vi "HFRR ADV v05.vi"() -> ()   [LabVIEW 2025] (continued)
      tunnel: w686 -> [w706 w859]
      tunnel: [w705 _] -> _
      frame No Error {
        n460 = stacked-sequence {
          tunnel: w706 -> [w730 _]
          tunnel: w702 -> [w729 _]
          tunnel: [w716 _] -> w705
          tunnel: [w715 _] -> w704
          tunnel: [w714 _] -> w703
          frame #0 {
            n461 = property class="Instr"(reference=w730, error in=w729) -> (reference out=w713:refnum<visa-resource-name>, error out=w728:errorcluster, "Serial Settings:Number of Bytes at Serial Port"=w709:u32)
            "Port 2" <- w709
            n462 = Greater?(x=w709, y=u32 23) -> (0:w711:bool)
            n463 = Not(x=w711) -> ()  [unwired: 1 out]
            n464 = case shown="True" w711 {
              tunnel: w713 -> [w745 w770]
              tunnel: w728 -> [w744 w771]
              tunnel: [w744 w773] -> w724
              tunnel: [w745 w772] -> w725
              frame False {
              }
              frame True {
                # "Out as Volts"
                n465 = local read "Residual Due"() -> (w769:string)
                n466 = while {
                  tunnel: [w813] -> w773
                  tunnel: [w812] -> w772
                  tunnel: w771 -> [w811]
                  tunnel: w770 -> [w810]
                  tunnel: [w807] -> _
                  shift-right: [w805] -> w768
                  shift-left: w769 -> [w804]
                  i -> [w807]
                  stop <- w808 stop-if-true
                  n467 = property class="Instr"(reference=w810, error in=w811) -> (reference out=w815:refnum<visa-resource-name>, error out=w814:errorcluster, "Serial Settings:Number of Bytes at Serial Port"=w806:u32)
                  n468 = VISA Read(VISA resource name=w815, byte count=w806, error in (no error)=w814) -> (VISA resource name out=w812:refnum<visa-resource-name>, read buffer=w803:string, error out=w813:errorcluster)  [unwired: 1 out]
                  n469 = Greater?(x=w806, y=u32 8) -> (0:w808:bool)
                  n470 = Concatenate Strings(w804, w803) -> (w805:string)
                }
                n471 = while {
                  shift-right: [w796] -> w752
                  shift-left: w768 -> [w801]
                  tunnel: [w795] -> w764 mode=indexing
                  tunnel: [w794] -> _
                  i -> [w794]
                  stop <- w798 stop-if-true
                  n472 = Match Pattern(string=w801, regular expression="*") -> (after substring=w799:string)  [unwired: 1 in, 3 out]
                  n473 = Match Pattern(string=w799, regular expression="&") -> (before substring=w795:string, after substring=w796:string, offset past match=w797:i32)  [unwired: 1 in, 1 out]
                  n474 = Less Than 0?(x=w797) -> (x < 0?=w798:bool)
                }
                n475 = Array Size(array=w764) -> (size(s)=w767:i32)
                n476 = local write "Residual Due"(w752) -> ()
                n477 = Decrement(x=w767) -> (x-1=w765:i32)
                n478 = Delete From Array(array=w764, length=1, index=w765) -> (array with subset deleted=w763:string[])  [unwired: 1 out]
                n479 = Array Size(array=w763) -> (size(s)=w751:i32)
                n480 = Decrement(x=w751) -> (x-1=w750:i32)
                n481 = while {
                  tunnel: w763 -> [w782] mode=indexing
                  tunnel: w750 -> [w781]
                  tunnel: [w779] -> w758 mode=indexing
                  tunnel: [w778] -> w757 mode=indexing
                  tunnel: [w777] -> w756 mode=indexing
                  tunnel: [w776] -> w755 mode=indexing
                  tunnel: [w775] -> w753 mode=indexing
                  tunnel: [w774] -> _
                  i -> [w774]
                  stop <- w780 stop-if-true
                  w791 = u32 0 ("length (rest)")
                  w790 = ";" ("regular expression")
                  n482 = Less Or Equal?(x=w781, y=w774) -> (x <= y?=w780:bool)
                  n483 = Match Pattern(string=w782, regular expression=w790) -> (before substring=w783:string, after substring=w784:string)  [unwired: 1 in, 2 out]
                  n484 = Match Pattern(string=w784, regular expression=w790) -> (before substring=w787:string, after substring=w785:string)  [unwired: 1 in, 2 out]
                  n485 = Decimal String To Number(string=w783, default (0L)=w791) -> (number=w779:u32)  [unwired: 1 in, 1 out]
                  n486 = Decimal String To Number(string=w787, default (0L)=w791) -> (number=w778:u32)  [unwired: 1 in, 1 out]
                  n487 = Match Pattern(string=w785, regular expression=w790) -> (before substring=w788:string, after substring=w786:string)  [unwired: 1 in, 2 out]
                  n488 = Decimal String To Number(string=w788, default (0L)=w791) -> (number=w777:u32)  [unwired: 1 in, 1 out]
                  n489 = Match Pattern(string=w786, regular expression=w790) -> (before substring=w789:string, after substring=w793:string)  [unwired: 1 in, 2 out]
                  n490 = Decimal String To Number(string=w789, default (0L)=w791) -> (number=w776:u32)  [unwired: 1 in, 1 out]
                  n491 = Decimal String To Number(string=w793, default (0L)=u8 0 ("length (rest)")) -> (number=w775:u8)  [unwired: 1 in, 1 out]
                }
                "Din" <- w753
                n492 = Bundle(w758, w757, w756, w755) -> (w760:cluster{u32[], u32[], u32[], u32[]})  [unwired: 1 in]
                n493 = Divide(x=w760, y=4095 ("length (rest)")) -> (x/y=w762:cluster{dbl[], dbl[], dbl[], dbl[]})
                n494 = Multiply(x=w762, y=sgl 3.32 ("Numeric")) -> (x*y=w754:cluster{dbl[], dbl[], dbl[], dbl[]})
                n495 = Unbundle(w754) -> (→"ECR":dbl[], →"Rtemp":dbl[], →"Air temp":dbl[], →"Ch3 2":dbl[])
              }
            }
            n496 = call "Elapsed Time10"("Time Target (s)"=2.0, "Reset"=w711, "Auto Reset"=FALSE) -> ("Time has Elapsed"=→"Port 2a":bool)  [unwired: 9 in, 7 out]
            n497 = local read "Due Com"() -> (w717:string[])
            n498 = Array Size(array=w717) -> (size(s)=w716:i32)
            n499 = Delete From Array(array=w717, length=1, index=0) -> (deleted portion=w720:string[], array with subset deleted=w721:string[])
            n500 = local write "Due Com"(w721) -> ()
            n501 = Index Array(array=w720, index=0) -> (element=w718:string)
            n502 = Not Equal?(x=w718, y="") -> (x != y?=w726:bool)
            n503 = case shown="True" w726 {
              tunnel: w725 -> [w732 w737]
              tunnel: [w732 w741] -> w715
              tunnel: w724 -> [w731 w736]
              tunnel: [w731 w739] -> w714
              tunnel: w718 -> [_ w735]
              tunnel: [_ w738] -> _
              frame False {
                # "DATA  WRITE LOOP"
              }
              frame True {
                n504 = Concatenate Strings(w735, "\r\n") -> (w734:string)
                n505 = VISA Write(VISA resource name=w737, write buffer=w734, error in (no error)=w736) -> (VISA resource name out=w741:refnum<visa-resource-name>, return count=w738:u32, error out=w740:errorcluster)
                n506 = flat-sequence {
                  tunnel: w740 -> [w742]
                  tunnel: [w742] -> w739
                  frame #0 {
                    n507 = Wait (ms)(milliseconds to wait=u32 5) -> ()  [unwired: 1 out]
                  }
                }
              }
            }
          }
          frame #1 {
            w824 = 10 ("y")
            w829 = 10 ("y")
            n508 = local read "Rtemp"() -> (w817:dbl[])
            n509 = local read "ecr buf"() -> (w818:dbl[])
            n510 = for {
              tunnel: w817 -> [w841] mode=indexing
              shift-right: [w842] -> w825
              shift-left: dbl[] [] ("temp buf 2") -> [w843]
              n511 = Build Array (concatenate)(w843, w841) -> (w844:dbl[])
              n512 = Equal To 0?(x=w841) -> (x = 0?=w845:bool)
              n513 = Select(t=w843, s=w845, f=w844) -> (s? t:f=w842:dbl[])
            }
            n514 = local read "ECR"() -> (w816:dbl[])
            n515 = Insert Into Array(array=w816, index=0, new element=w818) -> (w822:dbl[])
            n516 = local read "temp buf"() -> (w826:dbl[])
            n517 = Array Size(array=w822) -> (size(s)=w823:i32)
            n518 = Greater?(x=w823, y=w824) -> (0:w821:bool)
            n519 = case shown="True" w821 {
              tunnel: w822 -> [w834 w840]
              tunnel: w823 -> [_ w838]
              tunnel: w824 -> [_ w837]
              tunnel: [w834 w835] -> w819
              frame False {
              }
              frame True {
                n520 = Subtract(x=w838, y=w837) -> (x-y=w836:i32)
                n521 = Delete From Array(array=w840, length=w836, index=0) -> (array with subset deleted=w835:dbl[])  [unwired: 1 out]
              }
            }
            "ecr buf" <- w819
            n522 = Insert Into Array(array=w825, index=0, new element=w826) -> (w831:dbl[])
            n523 = Array Size(array=w831) -> (size(s)=w830:i32)
            n524 = Greater?(x=w830, y=w829) -> (0:w832:bool)
            n525 = case shown="True" w832 {
              tunnel: w831 -> [w846 w852]
              tunnel: w830 -> [_ w850]
              tunnel: w829 -> [_ w849]
              tunnel: [w846 w847] -> w828
              frame False {
              }
              frame True {
                n526 = Subtract(x=w850, y=w849) -> (x-y=w848:i32)
                n527 = Delete From Array(array=w852, length=w848, index=0) -> (array with subset deleted=w847:dbl[])  [unwired: 1 out]
              }
            }
            "temp buf" <- w828
          }
        }
      }
      frame Error {
        w867 = u16 0 items=["None", "XON/XOFF", "RTS/CTS", "XON/XOFF & RTS/CTS", "DTR/DSR", "XON/XOFF & DTR/DSR"] ("flow control (0:none)  2")
        w865 = u16 10 items=["1.0"=10, "1.5"=15, "2.0"=20] ("stop bits 2")
        w863 = u16 0 items=["None", "Odd", "Even", "Mark", "Space"] ("parity 2")
        w864 = u32 10000  # timeout (10sec)
        n528 = VISA Clear(VISA resource name=w859, error in (no error)=w856) -> (VISA resource name out=w858:refnum<visa-resource-name>, error out=w857:errorcluster)
        n529 = VISA Close(VISA resource name=w858, error in (no error)=w857) -> (error out=w860:errorcluster)
        n530 = call <vilib>:"Clear Errors.vi"("error in (no error)"=w860) -> ()  [unwired: 5 in, 2 out]
        n531 = local read "Com Port 2"() -> (w853:refnum<visa-resource-name>)
        "visa due" <- w853
        n532 = call-poly "VISA Configure Serial Port"("VISA resource name"=w853, "timeout (10sec)"=w864, "baud rate (9600)"=u32 250000 ("baud rate  2"), "data bits (8)"=u16 8 ("data bits  2"), "parity (0:none)"=w863, "stop bits (10: 1 bit)"=w865, "flow control (0:none)"=w867) -> ("VISA resource name out"=w868:refnum<visa-resource-name>, "error out"=w869:errorcluster)  [unwired: 7 in]
        n533 = flat-sequence {
          tunnel: w868 -> [w871]
          tunnel: w869 -> [w870]
          tunnel: [w871] -> w861
          tunnel: [w870] -> w854
          frame #0 {
            n534 = Wait (ms)(milliseconds to wait=u32 50) -> ()  [unwired: 1 out]
          }
        }
        "Residual Due" <- ""
        "Port 2 Error" <- w854
      }
    }
    n535 = local read "Quit"() -> (w680:bool)
    "Error Due" <- w688
  }
  n536 = property on="RUN" class="Bool (strict)"("Visible"=TRUE) -> ()  [unwired: 2 in, 2 out]
  n537 = while {
    tunnel: [w889] -> _
    tunnel: [w873] -> w38
    i -> [w889]
    stop <- w873 stop-if-true
    n538 = local read "conststatus"() -> (w877:dbl)
    n539 = local read "Main Tab"() -> (w875:T2)
    n540 = local read "EDIT"() -> (w895:bool)
    n541 = local read "Rate"() -> (w894:dbl)
    n542 = case shown="True" w895 {
      tunnel: [FALSE TRUE] -> w881
      frame False {
      }
      frame True {
      }
    }
    n543 = property on="Time slide" class="Slide (strict)"("Scale.Range:Maximum"=2500.0) -> ()  [unwired: 2 in, 2 out]
    n544 = Equal?(x=w875, y=T15."About" ("Main Tab")) -> (x = y?=w887:bool)
    n545 = Equal?(x=w877, y=0.0) -> (x = y?=w878:bool)
    n546 = Divide(x=1.0, y=w894) -> (x/y=w890:dbl)
    "Time 2" <- w890
    n547 = case shown="True" w878 {
      frame False {
      }
      frame True {
        # "C:\\WinDucom\\calibrate WO 2391.dcf"
        n548 = local write "Lan flag"(22) -> ()
        n549 = local write "conststatus"(10.0 ("rpm value : 2")) -> ()
        n550 = String To Path(string="C:\\LAB-IQ-NXT\\calibrate WO 2464.dcf") -> (path=w901:path)
        n551 = Open/Create/Replace File "Open File"(file path (use dialog)=w901) -> (refnum out=w899:refnum<file>)  [unwired: 5 in, 2 out]
        n552 = for {
          N: 23 -> [_]
          tunnel: w899 -> [w910]
          i -> [w904]
          (unwired) TRUE ("line mode (F)")
          n553 = Read from Text File "Read File"(file (use dialog)=w910) -> (text=w909:string)  [unwired: 3 in, 3 out]
          n554 = Match Pattern(string=w909, regular expression="]") -> (after substring=w907:string)  [unwired: 1 in, 3 out]
          n555 = String Subset(string=w909, offset (0)=5, length (rest)=10 ("length (rest)")) -> (substring=w902:string)
          n556 = Fract/Exp String To Number(string=w902) -> (number=w903:dbl)  [unwired: 3 in, 1 out]
          n557 = Match Pattern(string=w907, regular expression="-") -> (before substring=w905:string)  [unwired: 1 in, 3 out]
          n558 = case shown="18" w904 {
            tunnel: w903 -> [w913 w914 w915 w916 _ _ _ w921 w922 w923 w926 w927 w928 w929 w930 w931 w932 w935 w936 _ _ w939 _ _]
            tunnel: w905 -> [_ _ _ _ w917 w918 w919 _ _ _ _ _ _ _ _ _ _ _ _ w937 w938 _ w940 _]
            frame 0 {
              n559 = local write "FRIC. FORCE :"(w913) -> ()
            }
            frame 1 {
              n560 = local write "TEMPERATURE :"(w914) -> ()
            }
            frame 2 {
              n561 = local write "HUMIDITY:"(w915) -> ()
            }
            frame 3 {
              n562 = local write "AIR TEMPERATURE :"(w916) -> ()
            }
            frame 4 {
              n563 = local write "Com Port 1"(w917) -> ()
            }
            frame 5 {
              n564 = local write "Com Port 2"(w918) -> ()
              n565 = local write "visa due"(w918) -> ()
            }
            frame 6 {
              n566 = String To Path(string=w919) -> (path=w920:path)
              n567 = local write "File Path"(w920) -> ()
              "String" <- w919
            }
            frame 7 {
              n568 = local write "DISPLACEMENT :"(w921) -> ()
            }
            frame 8 {
              n569 = local write "STROKE GAIN :"(w922) -> ()
            }
            frame 9 {
              n570 = local read "Stroke PID Gains"() -> (w925:T8)
              n571 = Bundle By Name(cluster=w925, "Proportional Gain (Kc)"=w923) -> (w924:T8)
              n572 = local write "Stroke PID Gains"(w924) -> ()
            }
            frame 10 {
              n573 = local write "Language Selection"(w926) -> ()
            }
            frame 11 {
              n574 = local write "CH-POWER +"(w927) -> ()
            }
            frame 12 {
              n575 = local write "CH-POWER -"(w928) -> ()
            }
            frame 13 {
              n576 = local write "CH-HEATER"(w929) -> ()
            }
            frame 14 {
              n577 = local write "CH-HUMIDITY WET"(w930) -> ()
            }
            frame 15 {
              n578 = local write "CH-HUMIDITY DRY"(w931) -> ()
            }
            frame 16 {
              n579 = local read "Stroke PID Gains"() -> (w934:T8)
              n580 = Bundle By Name(cluster=w934, "Integral Time (Ti, min)"=w932) -> (w933:T8)
              n581 = local write "Stroke PID Gains"(w933) -> ()
            }
            frame 17 {
              n582 = local write "AIR TEMP INTERCEPT:"(w935) -> ()
            }
            frame 18 {
              n583 = local write "TEMP INTERCEPT:"(w936) -> ()
            }
            frame 19 {
              n584 = local write "S.NO"(w937) -> ()
            }
            frame 20 {
              n585 = local write "Com Port 3"(w938) -> ()
            }
            frame 21 {
              n586 = local write "LvdtOff"(w939) -> ()
            }
            frame 22 {
              n587 = local write "Humidity"(w940) -> ()
            }
            frame 23, Default {
            }
          }
        }
      }
    }
    n588 = Select(t=u32 2500 ("milliseconds to wait"), s=w887, f=u32 500 ("milliseconds to wait")) -> (s? t:f=w885:u32)
    n589 = Multiply(x=w890, y=w885) -> (x*y=w892:dbl)
    n590 = property on="FF Calibration g" class="WFGraph (strict)"("Visible"=w881) -> ()  [unwired: 2 in, 2 out]
    n591 = property on="Lift" class="Bool (strict)"("Visible"=w881) -> ()  [unwired: 2 in, 2 out]
    n592 = property on="Threshold" class="DigNum (strict)"("Visible"=w881) -> ()  [unwired: 2 in, 2 out]
    n593 = property on="Time slide" class="Slide (strict)"("Visible"=w881) -> ()  [unwired: 2 in, 2 out]
    n594 = call "Elapsed Time2"("Time Target (s)"=w892, "Auto Reset"=TRUE) -> ("Time has Elapsed"=w882:bool)  [unwired: 10 in, 7 out]
    n595 = case shown="True" w882 {
      frame False {
        # "79.77669138"
        # "2.3554"
        n596 = local read "FRIC. FORCE :"() -> (w945:dbl)
        n597 = local read "FF cal val"() -> (w942:dbl[])
        n598 = Multiply(x=w945, y=79.77669138) -> (x*y=w944:dbl)
        n599 = Multiply(x=w942, y=w944) -> (x*y=→"FF Calibration g":dbl[])
        "Err Count" <- 0 ("y")
      }
      frame True {
        n600 = stacked-sequence {
          frame #0 {
            n601 = stacked-sequence {
              frame #0 {
                "Lift" <- TRUE ("Lift")
              }
            }
          }
          frame #1 {
            w957 = 2500 ("y")
            n602 = local read "RUN"() -> (w949:bool)
            n603 = local read "FF1"() -> (w952:dbl[])
            n604 = case shown="False" w949 {
              frame False {
                n605 = local write "Frequency"(0.0 ("Frequency")) -> ()
              }
              frame True {
              }
            }
            n606 = Array Size(array=w952) -> (size(s)=w951:i32)
            n607 = local read "Ch1"() -> (w948:dbl[])
            "Waveform Chart 2" <- w948
            n608 = call-poly <vilib>:"Mean.vi"("X"=w948) -> ("mean"=→"Raw Mean":dbl)  [unwired: 1 out]
            n609 = Insert Into Array(array=w952, index=w951, new element=w948) -> (w954:dbl[])
            n610 = Array Size(array=w954) -> (size(s)=w958:i32)
            n611 = Subtract(x=w958, y=w957) -> (x-y=w956:i32)
            n612 = Greater?(x=w958, y=w957) -> (0:w959:bool)
            n613 = case shown="True" w959 {
              tunnel: w956 -> [_ w963]
              tunnel: [w961 w965] -> w950
              tunnel: w954 -> [w961 w964]
              frame False {
              }
              frame True {
                n614 = Delete From Array(array=w964, length=w963, index=0) -> (array with subset deleted=w965:dbl[])  [unwired: 1 out]
                "Numeric" <- w963
              }
            }
            "FF1" <- w950
            "PID Ref" <- TRUE ("PID Ref")
          }
          frame #2 {
          }
          frame #3 {
            w973 = 0.0 ("lower limit")
            # "CONVERT TO N"
            # "DATA PROCESSING"
            # "115 mV/N"
            n615 = local read "RH Numeric:"() -> (w967:dbl)
            n616 = local read "HUMIDITY:"() -> (w968:dbl)
            n617 = local read "temp buf"() -> (w1031:dbl[])
            n618 = local read "Air temp"() -> (w1029:dbl[])
            n619 = local read "ecr buf"() -> (w990:dbl[])
            n620 = local read "Fric Val"() -> (w1035:dbl[])
            n621 = case shown="True" "Boolean 5" {
              frame False {
              }
              frame True {
                n622 = local write "Boolean 5"(FALSE) -> ()
                n623 = local write "Captured Values"(dbl[][] [] ("Captured Values")) -> ()
                n624 = local write "Best Fit"(dbl[] [] ("Best Fit")) -> ()
              }
            }
            n625 = local read "TEMPERATURE :"() -> (w1012:dbl)
            n626 = call-poly <vilib>:"Mean.vi"("X"=w990) -> ("mean"=w987:dbl)  [unwired: 1 out]
            n627 = call-poly <vilib>:"Mean.vi"("X"=w1029) -> ("mean"=w997:dbl)  [unwired: 1 out]
            "Raw air temp" <- w997
            n628 = call-poly <vilib>:"Mean.vi"("X"=w1031) -> ("mean"=w999:dbl)  [unwired: 1 out]
            "Raw specimen temp" <- w999
            n629 = local read "TEMP INTERCEPT:"() -> (w1004:dbl)
            n630 = Multiply(x=w967, y=w968) -> (x*y=→"Humidity ( %RH )" →"Hum" →"Hum 2":dbl)
            n631 = Multiply(x=w1035, y=1.0) -> (x*y=w1036:dbl[])
            n632 = local read "FRIC. FORCE :"() -> (w1028:dbl)
            n633 = Multiply(x=w999, y=w1012) -> (x*y=w993:dbl)
            n634 = local read "AIR TEMPERATURE :"() -> (w1013:dbl)
            n635 = local read "RUN"() -> (w1025:bool)
            n636 = Add(x=w997, y="Offset Air Temp") -> (x+y=w992:dbl)
            n637 = local read "AIR TEMP INTERCEPT:"() -> (w1009:dbl)
            n638 = case shown="0, Default" "Calibrating" {
              tunnel: w999 -> [w1055 _]
              tunnel: [w1055 w1056] -> w998
              tunnel: w997 -> [_ w1056]
              frame 0, Default {
              }
              frame 1 {
              }
            }
            n639 = Multiply(x=w987, y="ECR_Gain") -> (x*y=w986:dbl)
            n640 = Add(x=w993, y=w1004) -> (x+y=w1010:dbl)
            n641 = Multiply(x=w1028, y=79.77669138) -> (x*y=w1026:dbl)
            n642 = Select(t=0.01 ("FF fil1"), s=w1025, f=0.1 ("FF fil1")) -> (s? t:f=w1021:dbl)
            n643 = local read "ecr"() -> (w981:dbl)
            n644 = Multiply(x=w992, y=w1013) -> (x*y=w994:dbl)
            n645 = Multiply(x=w1036, y=w1026) -> (x*y=w1033:dbl[])
            n646 = Multiply(x=w986, y=0.2) -> (x*y=w979:dbl)
            n647 = Multiply(x=0.8, y=w981) -> (x*y=w980:dbl)
            n648 = call <vilib>:"Mean PtByPt.vi"("x"=w1010, "sample length"=10) -> ("mean"=w969:dbl)  [unwired: 2 in, 1 out]
            "TEMP 2" <- w969
            "TEMP 3" <- w969
            n649 = local read "AIR TEMP"() -> (w1018:dbl)
            n650 = Add(x=w994, y=w1009) -> (x+y=w1011:dbl)
            n651 = call-poly <vilib>:"Mean.vi"("X"=w1033) -> ("mean"=w1034:dbl)  [unwired: 1 out]
            n652 = Add(x=w979, y=w980) -> (x+y=w978:dbl)
            n653 = Subtract(x=1.0 ("y"), y=w1021) -> (x-y=w1019:dbl)
            n654 = local write "TEMP"(w969) -> ()
            n655 = Multiply(x=w1019, y=w1018) -> (x*y=w1017:dbl)
            n656 = Multiply(x=w1011, y=w1021) -> (x*y=w1022:dbl)
            n657 = Not A Number/Path/Refnum?(number/path/refnum=w978) -> (NaN/Path/Refnum?=w988:bool)
            n658 = Subtract(x=w1033, y=w1034) -> (x-y=w1003:dbl[])
            n659 = local read "FRICVALZ"() -> (w1043:dbl)
            n660 = case shown="True" "Boolean 4" {
              tunnel: w998 -> [_ w1062]
              tunnel: "Standard Temp. ( °c )" -> [_ w1061]
              frame False {
              }
              frame True {
                n661 = Build Array(w1061, w1062) -> (w1060:dbl[])
                n662 = local write "Boolean 4"(FALSE ("Boolean 4")) -> ()
                n663 = local read "Captured Values"() -> (w1059:dbl[][])
                n664 = Build Array (concatenate)(w1059, w1060) -> (w1057:dbl[][])
                n665 = local write "Captured Values"(w1057) -> ()
              }
            }
            n666 = Or(x="FRICVALZ 3", y="FRICVALZ 2") -> (x .or. y?=w971:bool)
            n667 = Add(x=w1022, y=w1017) -> (x+y=w1015:dbl)
            n668 = Absolute Value(x=w1003) -> (abs(x)=w1038:dbl[])
            n669 = call-poly <vilib>:"RMS.vi"("X"=w1003) -> ("rms value"=w1002:dbl)  [unwired: 1 out]
            n670 = Select(t=0.0, s=w988, f=w978) -> (s? t:f=w985:dbl)
            n671 = call-poly <vilib>:"Mean.vi"("X"=w1038) -> ()  [unwired: 2 out]
            n672 = local read "FF 2"() -> (w1045:dbl)
            n673 = case shown="True" w971 {
              tunnel: w1002 -> [_ w1067]
              frame False {
              }
              frame True {
                w1066 = FALSE ("FRICVALZ")
                n674 = local write "FRICVALZ 3"(w1066) -> ()
                n675 = local write "FRICVALZ 2"(w1066) -> ()
                "FRICVALZ" <- w1067
              }
            }
            n676 = Subtract(x=w1002, y=w1043) -> (x-y=w1037:dbl)
            n677 = Not A Number/Path/Refnum?(number/path/refnum=w1015) -> (NaN/Path/Refnum?=w1016:bool)
            n678 = In Range and Coerce(upper limit=100.0, x=w985, lower limit=w973) -> ()  [unwired: 2 out]
            n679 = Select(t=0.0, s=w1016, f=w1015) -> (s? t:f=w975:dbl)
            "AIR TEMP" <- w975
            n680 = Multiply(x=w1037, y=0.1 ("FF fil1")) -> (x*y=w1049:dbl)
            n681 = Multiply(x=0.9 ("FF fil2"), y=w1045) -> (x*y=w1048:dbl)
            n682 = call "Elapsed Time11"("Time Target (s)"=1.0) -> ("Time has Elapsed"=w977:bool)  [unwired: 11 in, 7 out]
            n683 = Add(x=w1049, y=w1048) -> (x+y=w972:dbl)
            "FF 2" <- w972
            "FF 4" <- w972
            n684 = local read "NORMAL LOAD"() -> (w1032:dbl)
            n685 = case shown="True" w977 {
              tunnel: w975 -> [_ w1051]
              frame False {
              }
              frame True {
                "AirT" <- w1051
              }
            }
            n686 = local read "TEMP"() -> (w1042:dbl)
            n687 = Not A Number/Path/Refnum?(number/path/refnum=w972) -> (NaN/Path/Refnum?=w1040:bool)
            n688 = Divide(x=w972, y=w1032) -> (x/y=w1005:dbl)
            n689 = Not A Number/Path/Refnum?(number/path/refnum=w1042) -> (NaN/Path/Refnum?=w1041:bool)
            n690 = Compound Arithmetic op=OR(w1041, w1040) -> (w1039:bool)
            n691 = Not A Number/Path/Refnum?(number/path/refnum=w1005) -> (NaN/Path/Refnum?=w1007:bool)
            n692 = case shown="True" w1039 {
              frame False {
              }
              frame True {
                n693 = local write "TEMP"(0.0 ("TEMP")) -> ()
                n694 = local write "FF 2"(0.0 ("FF 2")) -> ()
                n695 = local write "reinit"(TRUE ("reinit")) -> ()
              }
            }
            n696 = Select(t=0.0, s=w1007, f=w1005) -> (s? t:f=→"COF 2":dbl)
            "ecr" <- w973
          }
          frame #4 {
            n697 = flat-sequence {
              frame #0 {
                n698 = Wait (ms)(milliseconds to wait=u32 100) -> ()  [unwired: 1 out]
              }
              frame #1 {
                n699 = local write "Lift"(FALSE ("Lift")) -> ()
              }
            }
            n700 = case shown="True" "Boolean 6" {
              frame False {
              }
              frame True {
                n701 = local write "Boolean 6"(FALSE ("Boolean 6")) -> ()
                n702 = local read "Captured Values"() -> (w1078:dbl[][])
                n703 = Index Array(array=w1078, index (col) #1=0 ("disabled index (col)"), index (col) #2=1 ("index (col)")) -> (element #1=w1076:dbl[], element #2=w1074:dbl[])  [unwired: 2 in]
                n704 = call <vilib>:"Linear Fit.vi"("Y"=w1076, "X"=w1074) -> ("Best Linear Fit"=→"Best Fit":dbl[], "slope"=w1070:dbl, "intercept"=w1069:dbl)  [unwired: 9 in, 2 out]
                "Slope" <- w1070
                "Intercept" <- w1069
                n705 = local read "Calibrating"() -> (w1071:u16)
                n706 = case shown="1" w1071 {
                  tunnel: w1070 -> [w1080 w1082]
                  tunnel: w1069 -> [w1079 w1081]
                  frame 0, Default {
                    n707 = local write "TEMPERATURE :"(w1080) -> ()
                    n708 = local write "TEMP INTERCEPT:"(w1079) -> ()
                  }
                  frame 1 {
                    n709 = local write "AIR TEMPERATURE :"(w1082) -> ()
                    n710 = local write "AIR TEMP INTERCEPT:"(w1081) -> ()
                  }
                }
              }
            }
          }
        }
      }
    }
    n711 = Wait (ms)(milliseconds to wait=u32 50) -> ()  [unwired: 1 out]
    n712 = local read "Quit"() -> (w873:bool)
    "Rate" <- 2500.0 ("No of Samples")
    "Humid Last buf" <- dbl[] [0.0, 0.0, 0.0, 0.0] ("Humid Last buf")
  }
  n713 = while {
    tunnel: w43 -> [_]
    tunnel: [w1112] -> _
    tunnel: [w1087] -> w40
    i -> [w1112]
    stop <- w1087 stop-if-true
    # "C:\\LAB-IQ-NXT\\Scar View.exe"
    n714 = local read "OK Button 16"() -> (w1101:bool)
    n715 = flat-sequence {
      frame #0 {
        n716 = stacked-sequence {
          frame #0 {
            n717 = local read "EDIT"() -> (w1766:bool)
            n718 = case shown="True" w1766 {
              tunnel: [u8 2 ("Disabled") u8 0 ("Disabled")] -> _
              frame False {
                w1768 = FALSE
                n719 = local write "Password"("") -> ()
                n720 = property on="SrvM CP" class="Bool (strict)"("Visible"=w1768) -> ()  [unwired: 2 in, 2 out]
                n721 = property on="message" class="Str"("Visible"=w1768) -> ()  [unwired: 2 in, 2 out]
                n722 = local write "x = y?"(w1768) -> ()
                n723 = property on="Password" class="Str"("Visible"=w1768) -> ()  [unwired: 2 in, 2 out]
                n724 = property on="ENTER THE NEW PASSWORD" class="Str"("Visible"=w1768) -> ()  [unwired: 2 in, 2 out]
                n725 = property on="ENTER CURRENT PASSWORD" class="Str"("Visible"=w1768) -> ()  [unwired: 2 in, 2 out]
                n726 = local write "SrvM CP"(w1768) -> ()
              }
              frame True {
                w1771 = TRUE
                n727 = property on="SrvM CP" class="Bool (strict)"("Visible"=w1771) -> ()  [unwired: 2 in, 2 out]
                n728 = property on="Password" class="Str"("Visible"=w1771) -> ()  [unwired: 2 in, 2 out]
              }
            }
            "dipl pwd" <- "@143$\n" ("dipl pwd")
          }
          frame #1 {
            # "Gain password"
            n729 = String To Byte Array(string="ENTER CURRENT PASSWORD") -> (unsigned byte array=w1776:u8[])
            n730 = Search 1D Array(1D array=w1776, element=u8 10) -> (index of element=w1779:i32)  [unwired: 1 in]
            n731 = Index Array(array=w1776, index=w1779) -> (element=w1775:u8)
            n732 = Equal?(x=w1775, y=10) -> (x = y?=w1773:bool)
            n733 = case shown="True" w1773 {
              frame False {
                n734 = property on="ENTER THE NEW PASSWORD" class="Str"("Visible"=FALSE) -> ()  [unwired: 2 in, 2 out]
              }
              frame True {
                # "password"
                # "change password logic"
                n735 = local read "ENTER CURRENT PASSWORD"() -> (w1792:string)
                n736 = local read "dipl pwd"() -> (w1786:string)
                n737 = String To Byte Array(string=w1792) -> (unsigned byte array=w1794:u8[])
                n738 = String To Byte Array(string=w1786) -> (unsigned byte array=w1787:u8[])
                n739 = Array Size(array=w1794) -> (size(s)=w1791:i32)
                n740 = Array Size(array=w1787) -> (size(s)=w1789:i32)
                n741 = for {
                  N: w1791 -> [_]
                  tunnel: w1794 -> [w1818]
                  tunnel: [w1816] -> w1795 mode=indexing
                  tunnel: w1791 -> [w1810]
                  i -> [w1811]
                  n742 = Decrement(x=w1810) -> (x-1=w1808:i32)
                  n743 = Equal?(x=w1811, y=w1808) -> (x = y?=w1809:bool)
                  n744 = Index Array(array=w1818, index=w1811) -> (element=w1812:u8)
                  n745 = Number To Decimal String(number=w1812) -> (decimal integer string=w1817:string)  [unwired: 1 in]
                  n746 = Select(t="", s=w1809, f="\r") -> (s? t:f=w1814:string)
                  n747 = Concatenate Strings(w1817, w1814) -> (w1816:string)
                }
                n748 = for {
                  N: w1789 -> [_]
                  tunnel: w1787 -> [w1806]
                  tunnel: [w1804] -> w1788 mode=indexing
                  tunnel: w1789 -> [w1801]
                  i -> [w1802]
                  n749 = Decrement(x=w1801) -> (x-1=w1800:i32)
                  n750 = Equal?(x=w1802, y=w1800) -> (x = y?=w1799:bool)
                  n751 = Index Array(array=w1806, index=w1802) -> (element=w1805:u8)
                  n752 = Number To Decimal String(number=w1805) -> (decimal integer string=w1803:string)  [unwired: 1 in]
                  n753 = Select(t="", s=w1799, f="\r") -> (s? t:f=w1796:string)
                  n754 = Concatenate Strings(w1803, w1796) -> (w1804:string)
                }
                n755 = local read "string"() -> (w1793:string)
                n756 = Concatenate Strings(w1788) -> (w1782:string)
                n757 = Concatenate Strings(w1793) -> (w1790:string)
                n758 = Concatenate Strings(w1795) -> (w1783:string)
                n759 = Equal?(x=w1783, y=w1790) -> (x = y?=w1785:bool)
                n760 = Equal?(x=w1783, y=w1782) -> (x = y?=w1781:bool)
                n761 = Or(x=w1785, y=w1781) -> (x .or. y?=w1784:bool)
                n762 = case shown="True" w1784 {
                  frame False {
                  }
                  frame True {
                    n763 = property on="ENTER THE NEW PASSWORD" class="Str"("Visible"=TRUE) -> ()  [unwired: 2 in, 2 out]
                  }
                }
              }
            }
          }
          frame #2 {
            n764 = String To Byte Array(string="ENTER THE NEW PASSWORD") -> (unsigned byte array=w1821:u8[])
            n765 = Search 1D Array(1D array=w1821, element=u8 10) -> (index of element=w1825:i32)  [unwired: 1 in]
            n766 = Index Array(array=w1821, index=w1825) -> (element=w1823:u8)
            n767 = Equal?(x=w1823, y=10) -> (x = y?=w1820:bool)
            n768 = case shown="False" w1820 {
              frame False {
              }
              frame True {
                n769 = local write "EDIT"(FALSE) -> ()
                n770 = local write "SrvM CP"(FALSE) -> ()
                n771 = local read "ENTER THE NEW PASSWORD"() -> (w1828:string)
                n772 = String To Byte Array(string=w1828) -> (unsigned byte array=w1833:u8[])
                n773 = Array Size(array=w1833) -> (size(s)=w1830:i32)
                n774 = for {
                  N: w1830 -> [_]
                  tunnel: w1833 -> [w1846]
                  tunnel: [w1843] -> w1835 mode=indexing
                  tunnel: w1830 -> [w1838]
                  i -> [w1836]
                  n775 = Decrement(x=w1838) -> (x-1=w1839:i32)
                  n776 = Equal?(x=w1836, y=w1839) -> (x = y?=w1840:bool)
                  n777 = Index Array(array=w1846, index=w1836) -> (element=w1845:u8)
                  n778 = Number To Decimal String(number=w1845) -> (decimal integer string=w1844:string)  [unwired: 1 in]
                  n779 = Select(t="", s=w1840, f="\r") -> (s? t:f=w1837:string)
                  n780 = Concatenate Strings(w1844, w1837) -> (w1843:string)
                }
                n781 = local read "file path"() -> (w1827:path)
                n782 = Concatenate Strings(w1835) -> (w1829:string)
                n783 = Delete(path (use dialog)=w1827) -> (deleted path=w1831:path)  [unwired: 4 in, 2 out]
                n784 = call <vilib>:"Write Characters To File.vi"("append to file? (new file:F)"=FALSE, "character string"=w1829, "file path (dialog if empty)"=w1831) -> ()  [unwired: 2 in, 1 out]
              }
            }
          }
          frame #3 {
            n785 = case shown="True" "SrvM CP" {
              frame False {
                w1849 = ""
                n786 = local write "ENTER CURRENT PASSWORD"(w1849) -> ()
                n787 = local write "ENTER THE NEW PASSWORD"(w1849) -> ()
                n788 = property on="ENTER CURRENT PASSWORD" class="Str"("Visible"=FALSE) -> ()  [unwired: 2 in, 2 out]
              }
              frame True {
                n789 = property on="ENTER THE NEW PASSWORD" class="Str"() -> ("Visible"=w1850:bool)  [unwired: 2 in, 2 out]
                n790 = Not(x=w1850) -> (.not. x?=w1851:bool)
                n791 = property on="ENTER CURRENT PASSWORD" class="Str"("Visible"=w1851) -> ()  [unwired: 2 in, 2 out]
              }
            }
          }
          frame #4 {
            n792 = String To Byte Array(string="Password") -> (unsigned byte array=w1858:u8[])
            n793 = Search 1D Array(1D array=w1858, element=u8 10) -> (index of element=w1856:i32)  [unwired: 1 in]
            n794 = Index Array(array=w1858, index=w1856) -> (element=w1857:u8)
            n795 = Equal?(x=w1857, y=10) -> (x = y?=w1853:bool)
            n796 = case shown="True" w1853 {
              frame False {
              }
              frame True {
                # "password"
                # "password"
                n797 = local read "Password"() -> (w1871:string)
                n798 = String To Byte Array(string=w1871) -> (unsigned byte array=w1874:u8[])
                n799 = String To Byte Array(string="@143$\n") -> (unsigned byte array=w1860:u8[])
                n800 = Array Size(array=w1874) -> (size(s)=w1869:i32)
                n801 = Array Size(array=w1860) -> (size(s)=w1865:i32)
                n802 = for {
                  N: w1869 -> [_]
                  tunnel: w1874 -> [w1891]
                  tunnel: [w1889] -> w1875 mode=indexing
                  tunnel: w1869 -> [w1886]
                  i -> [w1887]
                  n803 = Decrement(x=w1886) -> (x-1=w1885:i32)
                  n804 = Index Array(array=w1891, index=w1887) -> (element=w1890:u8)
                  n805 = Equal?(x=w1887, y=w1885) -> (x = y?=w1884:bool)
                  n806 = Number To Decimal String(number=w1890) -> (decimal integer string=w1888:string)  [unwired: 1 in]
                  n807 = Select(t="", s=w1884, f="\r") -> (s? t:f=w1881:string)
                  n808 = Concatenate Strings(w1888, w1881) -> (w1889:string)
                }
                n809 = for {
                  N: w1865 -> [_]
                  tunnel: w1860 -> [w1902]
                  tunnel: [w1900] -> w1863 mode=indexing
                  tunnel: w1865 -> [w1897]
                  i -> [w1898]
                  n810 = Decrement(x=w1897) -> (x-1=w1896:i32)
                  n811 = Index Array(array=w1902, index=w1898) -> (element=w1901:u8)
                  n812 = Equal?(x=w1898, y=w1896) -> (x = y?=w1895:bool)
                  n813 = Number To Decimal String(number=w1901) -> (decimal integer string=w1899:string)  [unwired: 1 in]
                  n814 = Select(t="", s=w1895, f="\r") -> (s? t:f=w1892:string)
                  n815 = Concatenate Strings(w1899, w1892) -> (w1900:string)
                }
                n816 = local read "file path"() -> (w1859:path)
                n817 = call <vilib>:"Read Characters From File.vi"("file path (dialog if empty)"=w1859) -> ("character string"=w1873:string)  [unwired: 5 in, 3 out]
                "string" <- w1873
                n818 = flat-sequence {
                  tunnel: [w1876] -> w1870
                  frame #0 {
                    w1876 = ""
                    n819 = local write "Password"(w1876) -> ()
                  }
                }
                n820 = Concatenate Strings(w1863) -> (w1864:string)
                n821 = Concatenate Strings(w1873) -> (w1872:string)
                n822 = Concatenate Strings(w1875) -> (w1867:string)
                n823 = Equal?(x=w1867, y=w1872) -> (x = y?=w1862:bool)
                n824 = Equal?(x=w1867, y=w1864) -> (x = y?=w1868:bool)
                n825 = Or(x=w1862, y=w1868) -> (x .or. y?=w1861:bool)
                "x = y?" <- w1861
                n826 = case shown="False" w1861 {
                  selector: w1861 -> [w1878 _]
                  tunnel: w1870 -> [_ _]
                  frame False {
                    n827 = And(x=w1878, y=TRUE ("Visible")) -> (x .and. y?=w1879:bool)
                    n828 = property on="message" class="Str"("Visible"=w1879) -> ()  [unwired: 2 in, 2 out]
                  }
                  frame True {
                    n829 = property on="message" class="Str"("Visible"=FALSE) -> ()  [unwired: 2 in, 2 out]
                  }
                }
              }
            }
          }
        }
        n830 = local read "x = y?"() -> (w1718:bool)
        n831 = local read "HUMIDITY: 2"() -> (w1720:dbl)
        n832 = local read "HUMIDITY:"() -> (w1719:dbl)
        n833 = property on="Port 2 Error" class="Clust (strict)"("Visible"="EDIT") -> ()  [unwired: 2 in, 2 out]
        n834 = property on="Port 1 Error" class="Clust (strict)"("Visible"="EDIT") -> ()  [unwired: 2 in, 2 out]
        n835 = case shown="True" "SrvM CP 2" {
          frame False {
          }
          frame True {
            n836 = local write "SrvM CP 2"(FALSE ("SrvM CP 2")) -> ()
            n837 = local read "HUMIDITY: 2"() -> (w1759:dbl)
            n838 = local read "TEMP INTERCEPT: 2"() -> (w1758:dbl)
            n839 = local read "DISPLACEMENT : 4"() -> (w1762:dbl)
            n840 = local read "TEMPERATURE : 2"() -> (w1761:dbl)
            n841 = local read "STROKE GAIN : 2"() -> (w1763:dbl)
            n842 = local read "FRIC. FORCE : 2"() -> (w1764:dbl)
            n843 = local read "AIR TEMP INTERCEPT: 2"() -> (w1757:dbl)
            n844 = local read "AIR TEMPERATURE : 2"() -> (w1760:dbl)
            n845 = local write "HUMIDITY:"(w1759) -> ()
            n846 = local write "AIR TEMP INTERCEPT:"(w1758) -> ()
            n847 = local write "TEMPERATURE :"(w1761) -> ()
            n848 = local write "FRIC. FORCE :"(w1764) -> ()
            n849 = local write "STROKE GAIN :"(w1763) -> ()
            n850 = local write "DISPLACEMENT :"(w1762) -> ()
            n851 = local write "AIR TEMPERATURE :"(w1760) -> ()
            n852 = local write "TEMP INTERCEPT:"(w1757) -> ()
          }
        }
        n853 = case shown="True" "SAVE" {
          frame False {
          }
          frame True {
            n854 = stacked-sequence {
              seq-local: [w1919 _ _] -> [_ w2078 _]
              frame #0 {
                (unwired) i16 5 ("precision (6)")
                # "[CH1]    - FF\n[CH2]   - TEMPERATURE\n[CH3]    - Humidity\n[CH4]    - AIR TEMP\n[CH5]\\- Visa Uno\n[CH6] \\- Visa Due\n[CH7]  \\- file path\n[CH8]   - Displacement Gain\n[CHA]   - Stroke Gain\n[CHB]   - Stroke PID Gain\n[CHC]   -Language Selection\n[CHD]   -Power +\n[CHE]   -Power_\n[CHF]   -Heater\n[CHG]   -Humidity Wet\n[CHH]   -Humidity Dry\n[CHI]   -Integral Time"
                n855 = local read "Stroke PID Gains"() -> (w1970:T8)
                n856 = Unbundle By Name(w1970) -> ("Proportional Gain (Kc)"=w1969:dbl, "Integral Time (Ti, min)"=w1911:dbl)
                n857 = Number To Fractional String(number=w1911, width (-)=i16 10 ("precision (6)"), precision (6)=i16 5) -> (F-format string=w1915:string)  [unwired: 1 in]
                n858 = local read "Language Selection"() -> (w1967:enum16{"English", "Russian"})
                n859 = local read "CH-HUMIDITY WET"() -> (w1925:u16)
                n860 = local read "CH-HUMIDITY DRY"() -> (w1922:u16)
                n861 = local read "STROKE GAIN :"() -> (w1903:dbl)
                n862 = local read "CH-POWER +"() -> (w1934:u16)
                n863 = local read "CH-POWER -"() -> (w1931:u16)
                n864 = local read "CH-HEATER"() -> (w1928:u16)
                n865 = local read "AIR TEMPERATURE :"() -> (w1906:dbl)
                n866 = Concatenate Strings("[CHI]" ("string"), w1915, "-Integral Time " ("string"), "\r") -> (w1912:string)
                n867 = local read "DISPLACEMENT :"() -> (w1904:dbl)
                n868 = local read "TEMPERATURE :"() -> (w1907:dbl)
                n869 = local read "FRIC. FORCE :"() -> (w1908:dbl)
                n870 = local read "HUMIDITY:"() -> (w1905:dbl)
                n871 = Path To String(path="File Path") -> (string=w1992:string)
                n872 = Number To Fractional String(number=w1903, width (-)=i16 10 ("precision (6)"), precision (6)=i16 5) -> (F-format string=w1983:string)  [unwired: 1 in]
                n873 = Number To Fractional String(number=w1969, width (-)=i16 10 ("precision (6)"), precision (6)=i16 5) -> (F-format string=w1971:string)  [unwired: 1 in]
                n874 = Number To Fractional String(number=w1967, width (-)=i16 10 ("precision (6)"), precision (6)=i16 5) -> (F-format string=w1963:string)  [unwired: 1 in]
                n875 = Number To Fractional String(number=w1934, width (-)=i16 10 ("precision (6)"), precision (6)=i16 5) -> (F-format string=w1957:string)  [unwired: 1 in]
                n876 = Number To Fractional String(number=w1931, width (-)=i16 10 ("precision (6)"), precision (6)=i16 5) -> (F-format string=w1954:string)  [unwired: 1 in]
                n877 = Number To Fractional String(number=w1928, width (-)=i16 10 ("precision (6)"), precision (6)=i16 5) -> (F-format string=w1949:string)  [unwired: 1 in]
                n878 = Number To Fractional String(number=w1925, width (-)=i16 10 ("precision (6)"), precision (6)=i16 5) -> (F-format string=w1946:string)  [unwired: 1 in]
                n879 = Number To Fractional String(number=w1922, width (-)=i16 10 ("precision (6)"), precision (6)=i16 5) -> (F-format string=w1941:string)  [unwired: 1 in]
                n880 = local read "Com Port 1"() -> (w1910:refnum<visa-resource-name>)
                n881 = local read "Com Port 2"() -> (w1909:refnum<visa-resource-name>)
                n882 = Concatenate Strings(w1992, "\\" ("string")) -> (w1991:string)
                n883 = Number To Fractional String(number=w1908, width (-)=i16 10 ("precision (6)"), precision (6)=i16 5) -> (F-format string=w2024:string)  [unwired: 1 in]
                n884 = Number To Fractional String(number=w1907, width (-)=i16 10 ("precision (6)"), precision (6)=i16 5) -> (F-format string=w2023:string)  [unwired: 1 in]
                n885 = Number To Fractional String(number=w1905, width (-)=i16 10 ("precision (6)"), precision (6)=i16 5) -> (F-format string=w2017:string)  [unwired: 1 in]
                n886 = Number To Fractional String(number=w1906, width (-)=i16 10 ("precision (6)"), precision (6)=i16 5) -> (F-format string=w2011:string)  [unwired: 1 in]
                n887 = Number To Fractional String(number=w1904, width (-)=i16 10 ("precision (6)"), precision (6)=i16 5) -> (F-format string=w1984:string)  [unwired: 1 in]
                n888 = Concatenate Strings("[CHA]" ("string"), w1983, "- Stroke Gain" ("string"), "\r") -> (w1977:string)
                n889 = Concatenate Strings("[CHB]" ("string"), w1971, "- Stroke PID Gain" ("string"), "\r") -> (w1968:string)
                n890 = Concatenate Strings("[CHC]" ("string"), w1963, "-Language Selection" ("string"), "\r") -> (w1960:string)
                n891 = Concatenate Strings("[CHD]" ("string"), w1957, "-Power +" ("string"), "\r") -> (w1939:string)
                n892 = Concatenate Strings("[CHG]" ("string"), w1946, "-Humidity Wet" ("string"), "\r") -> (w1936:string)
                n893 = Concatenate Strings("[CHH]" ("string"), w1941, "-Humidity Dry" ("string"), "\r") -> (w1935:string)
                n894 = Concatenate Strings("[CH1]" ("string"), w2024, " - FF" ("string"), "\r") -> (w2022:string)
                n895 = Concatenate Strings("[CH2]" ("string"), w2023, " - TEMPERATURE" ("string"), "\r") -> (w2021:string)
                n896 = Concatenate Strings("[CH3]" ("string"), w2017, " - Humidity" ("string"), "\r") -> (w2014:string)
                n897 = Concatenate Strings("[CH4]" ("string"), w2011, " - AIR TEMP" ("string"), "\r") -> (w2007:string)
                n898 = Concatenate Strings("[CH5]" ("string"), w1910, "- Visa Uno" ("string"), "\r") -> (w2000:string)
                n899 = Concatenate Strings("[CH6]" ("string"), w1909, "- Visa Due" ("string"), "\r") -> (w1995:string)
                n900 = Concatenate Strings("[CH7]" ("string"), w1991, "- file path" ("string"), "\r") -> (w1994:string)
                n901 = Concatenate Strings("[CH8]" ("string"), w1984, "- Displacement Gain" ("string"), "\r") -> (w1987:string)
                n902 = Concatenate Strings("[CHE]" ("string"), w1954, "-Power_" ("string"), "\r") -> (w1938:string)
                n903 = Concatenate Strings("[CHF]" ("string"), w1949, "-Heater" ("string"), "\r") -> (w1937:string)
                n904 = Concatenate Strings(w2022, w2021, w2014, w2007, w2000, w1995, w1994, w1987, w1977, w1968, w1960, w1939, w1938, w1937, w1936, w1935, w1912) -> (w1919:string)
                "gain" <- w1919
              }
              frame #1 {
                n905 = local read "TEMP INTERCEPT:"() -> (w2040:dbl)
                n906 = local read "Humidity"() -> (w2039:refnum<visa-resource-name>)
                n907 = local read "AIR TEMP INTERCEPT:"() -> (w2041:dbl)
                n908 = local read "LvdtOff"() -> (w2043:dbl)
                n909 = Number To Fractional String(number=w2040, width (-)=i16 10 ("precision (6)"), precision (6)=i16 5) -> (F-format string=w2066:string)  [unwired: 1 in]
                n910 = local read "Com Port 3"() -> (w2050:refnum<visa-resource-name>)
                n911 = Concatenate Strings("[CH7]" ("string"), w2039, "- Visa Humidity" ("string"), "\r") -> (w2035:string)
                n912 = Number To Fractional String(number=w2041, width (-)=i16 10 ("precision (6)"), precision (6)=i16 5) -> (F-format string=w2073:string)  [unwired: 1 in]
                n913 = Number To Fractional String(number=w2043, width (-)=i16 10 ("precision (6)"), precision (6)=i16 5) -> (F-format string=w2047:string)  [unwired: 1 in]
                n914 = Concatenate Strings("[CHK]" ("string"), w2066, "-TEMP INTERCEPT" ("string"), "\r") -> (w2062:string)
                n915 = Concatenate Strings("[SNO]" ("string"), "S.NO", "-" ("string"), "\r") -> (w2058:string)
                n916 = Concatenate Strings("[CHI]" ("string"), w2047, "-LVDT Position Offset" ("string"), "\r") -> (w2042:string)
                n917 = Concatenate Strings("[CHJ]" ("string"), w2073, "-AIR TEMP INTERCEPT" ("string"), "\r") -> (w2063:string)
                n918 = Concatenate Strings("[CHL]" ("string"), w2050, "- Visa humid" ("string"), "\r") -> (w2053:string)
                n919 = String To Path(string="C:\\LAB-IQ-NXT\\calibrate WO 2464.dcf") -> (path=w2051:path)
                n920 = Concatenate Strings(w2078, w2063, w2062, w2058, w2053, w2042, w2035) -> (w2077:string)
                n921 = call <vilib>:"Write Characters To File.vi"("append to file? (new file:F)"=FALSE, "character string"=w2077, "file path (dialog if empty)"=w2051) -> ()  [unwired: 2 in, 1 out]
              }
              frame #2 {
                n922 = local write "Lan flag"(0.0 ("Lan flag")) -> ()
                n923 = local write "conststatus"(0.0 ("rpm value : 2")) -> ()
                n924 = local write "SAVE"(FALSE ("OK Button 14")) -> ()
                n925 = local write "Re-Initialise"(TRUE ("Re-Initialise")) -> ()
              }
            }
          }
        }
        n926 = And(x="EDIT", y=w1718) -> (x .and. y?=w1716:bool)
        n927 = local read "DISPLACEMENT : 4"() -> (w1729:dbl)
        n928 = local read "TEMPERATURE : 2"() -> (w1727:dbl)
        n929 = local read "STROKE GAIN : 2"() -> (w1733:dbl)
        n930 = local read "DISPLACEMENT :"() -> (w1728:dbl)
        n931 = local read "FRIC. FORCE : 2"() -> (w1736:dbl)
        n932 = local read "TEMPERATURE :"() -> (w1725:dbl)
        n933 = local read "STROKE GAIN :"() -> (w1732:dbl)
        n934 = local read "FRIC. FORCE :"() -> (w1735:dbl)
        n935 = case shown="False" w1716 {
          tunnel: [u8 2 ("Disabled") u8 0 ("Disabled")] -> w1715
          tunnel: [w2083 TRUE ("Visible")] -> w1714
          frame False {
            w2083 = FALSE ("Visible")
            n936 = local write "EDIT 2"(w2083) -> ()
          }
          frame True {
          }
        }
        n937 = Subtract(x=w1720, y=w1719) -> (x-y=w1721:dbl)
        n938 = local read "AIR TEMPERATURE : 2"() -> (w1724:dbl)
        n939 = local read "AIR TEMPERATURE :"() -> (w1723:dbl)
        n940 = Divide(x=w1721, y=w1719) -> (x/y=w1743:dbl)
        n941 = Subtract(x=w1736, y=w1735) -> (x-y=w1734:dbl)
        n942 = Subtract(x=w1727, y=w1725) -> (x-y=w1726:dbl)
        n943 = Subtract(x=w1733, y=w1732) -> (x-y=w1731:dbl)
        n944 = Subtract(x=w1729, y=w1728) -> (x-y=w1730:dbl)
        n945 = Subtract(x=w1724, y=w1723) -> (x-y=w1722:dbl)
        n946 = Divide(x=w1734, y=w1735) -> (x/y=w1754:dbl)
        n947 = Divide(x=w1726, y=w1725) -> (x/y=w1747:dbl)
        n948 = Divide(x=w1731, y=w1732) -> (x/y=w1751:dbl)
        n949 = Divide(x=w1730, y=w1728) -> (x/y=w1750:dbl)
        n950 = Multiply(x=w1743, y=100.0) -> (x*y=→"HUMIDITY  Calibration Error":dbl)
        n951 = Divide(x=w1722, y=w1723) -> (x/y=w1746:dbl)
        n952 = Multiply(x=w1754, y=100.0) -> (x*y=→"FRIC. FORCE Calibration Error":dbl)
        n953 = Multiply(x=w1747, y=100.0) -> (x*y=→"TEMPERATURE  Calibration Error":dbl)
        n954 = Multiply(x=w1751, y=100.0) -> (x*y=→"STROKE Calibration Error":dbl)
        n955 = Multiply(x=w1750, y=100.0) -> (x*y=→"DISPLACEMENT  Calibration Error":dbl)
        n956 = property on="EDIT 2" class="Bool (strict)"("Visible"=w1714) -> ()  [unwired: 2 in, 2 out]
        n957 = property on="SAVE" class="Bool (strict)"("Visible"=w1714) -> ()  [unwired: 2 in, 2 out]
        n958 = property on="SrvM CP" class="Bool (strict)"("Disabled"=w1715) -> ()  [unwired: 2 in, 2 out]
        n959 = property on="visa due" class="CmbBox"("Disabled"=w1715) -> ()  [unwired: 2 in, 2 out]
        n960 = property on="LvdtOff" class="DigNum (strict)"("Disabled"=w1715) -> ()  [unwired: 2 in, 2 out]
        n961 = property on="File Path" class="Path"("Disabled"=w1715) -> ()  [unwired: 2 in, 2 out]
        n962 = Multiply(x=w1746, y=100.0) -> (x*y=→"AIR TEMPERATURE  Calibration Error":dbl)
        n963 = property on="Tab Control" class="TabCtl (strict)"("Visible"=w1714) -> ()  [unwired: 2 in, 2 out]
        n964 = property on="Language Selection" class="Enum (strict)"("Visible"=w1714) -> ()  [unwired: 2 in, 2 out]
        n965 = property on="Tab Control 7" class="TabCtl (strict)"("Disabled"=w1715) -> ()  [unwired: 2 in, 2 out]
        n966 = property on="AIR TEMP INTERCEPT:" class="DigNum (strict)"("Disabled"=w1715) -> ()  [unwired: 2 in, 2 out]
        n967 = property on="CH-POWER -" class="DigNum (strict)"("Disabled"=w1715) -> ()  [unwired: 2 in, 2 out]
        n968 = property on="CH-POWER +" class="DigNum (strict)"("Disabled"=w1715) -> ()  [unwired: 2 in, 2 out]
        n969 = property on="AIR TEMPERATURE :" class="DigNum (strict)"("Disabled"=w1715) -> ()  [unwired: 2 in, 2 out]
        n970 = property on="STROKE GAIN :" class="DigNum (strict)"("Disabled"=w1715) -> ()  [unwired: 2 in, 2 out]
        n971 = property on="SPEED OUT:" class="DigNum (strict)"("Disabled"=w1715) -> ()  [unwired: 2 in, 2 out]
        n972 = property on="CH-HUMIDITY DRY" class="DigNum (strict)"("Disabled"=w1715) -> ()  [unwired: 2 in, 2 out]
        n973 = property on="HUMIDITY:" class="DigNum (strict)"("Disabled"=w1715) -> ()  [unwired: 2 in, 2 out]
        n974 = property on="CH-HUMIDITY WET" class="DigNum (strict)"("Disabled"=w1715) -> ()  [unwired: 2 in, 2 out]
        n975 = property on="Stroke PID Gains" class="Clust (strict)"("Disabled"=w1715) -> ()  [unwired: 2 in, 2 out]
        n976 = property on="TEMPERATURE :" class="DigNum (strict)"("Disabled"=w1715) -> ()  [unwired: 2 in, 2 out]
        n977 = property on="DISPLACEMENT :" class="DigNum (strict)"("Disabled"=w1715) -> ()  [unwired: 2 in, 2 out]
        n978 = property on="CH-HEATER" class="DigNum (strict)"("Disabled"=w1715) -> ()  [unwired: 2 in, 2 out]
        n979 = property on="TEMP INTERCEPT:" class="DigNum (strict)"("Disabled"=w1715) -> ()  [unwired: 2 in, 2 out]
        n980 = property on="FRIC. FORCE :" class="DigNum (strict)"("Disabled"=w1715) -> ()  [unwired: 2 in, 2 out]
      }
    }
